vi "Elapsed time.vi"(9 "error in (no error)":errorcluster) -> (1 "error out":errorcluster, 2 "dt (sec)":dbl)   [LabVIEW 2013, in "Timing Lib.lvlib"]
doc: "Reentrant vi- will calculate elapsed times between instance calls"
uses:
  Timing Lib.lvlib
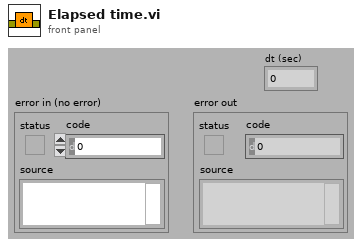
[diagram p1: front panel]
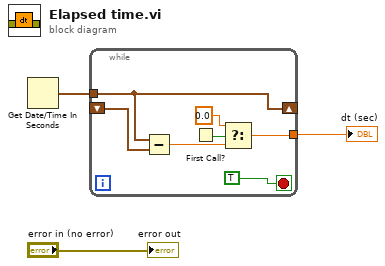
[diagram p0: block diagram]
diagram:
  n1 = Get Date/Time In Seconds() -> (seconds since 1Jan1904=w2:timestamp)
  n2 = while {
    shift-right: [w7] -> _
    shift-left: _ -> [w8]
    tunnel: w2 -> [w7]
    tunnel: [w5] -> w1
    stop <- TRUE stop-if-true
    n3 = Subtract(x=w7, y=w8) -> (x-y=w6:dbl)
    n4 = First Call?() -> (First Call?: T/F=w4:bool)
    n5 = Select(t=0.0, s=w4, f=w6) -> (s? t:f=w5:dbl)
  }
  "dt (sec)" <- w1
  "error out" <- "error in (no error)"
